vi "Speed Ramp.vi"(8 "Current Distance":dbl, 9 "Distance":dbl, 10 "End":dbl, 11 "Start":dbl) -> (3 "Speed":dbl)   [LabVIEW 2016]
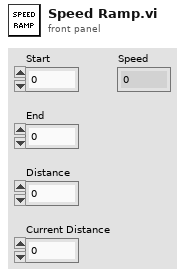
[diagram p1: front panel]
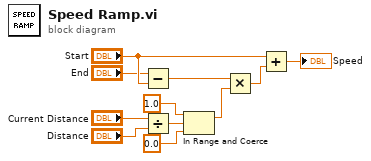
[diagram p0: block diagram]
diagram:
  n1 = Subtract(x="End", y="Start") -> (x-y=w7:dbl)
  n2 = Divide(x="Current Distance", y="Distance") -> (x/y=w4:dbl)
  n3 = In Range and Coerce(upper limit=1.0, x=w4, lower limit=0.0) -> (coerced(x)=w8:dbl)  [unwired: 1 out]
  n4 = Multiply(x=w7, y=w8) -> (x*y=w9:dbl)
  n5 = Add(x="Start", y=w9) -> (x+y=→"Speed":dbl)
